vi "ObtainCmdQueue.vi"(0 "queueName":string="default", 11 "error in (no error)":errorcluster) -> (4 "cmdRef":T1, 15 "error out":errorcluster)   [LabVIEW 2017, in "vsws.lvlib"]
uses:
  vsws.lvlib
  cmdRef.ctl
  cmd.ctl
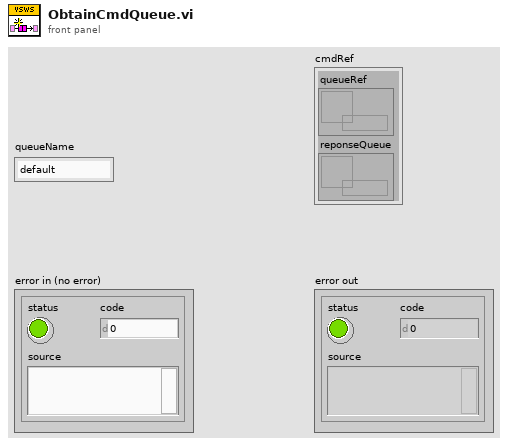
[diagram p1: front panel]
types:
  T1 = typedef "vsws.lvlib/cmdRef.ctl" = cluster{"queueRef":refnum<queue>, "reponseQueue":refnum<queue>}
  T2 = typedef "vsws.lvlib/cmd.ctl" = cluster{"postdata":string, "reponseQueue":refnum<queue>}
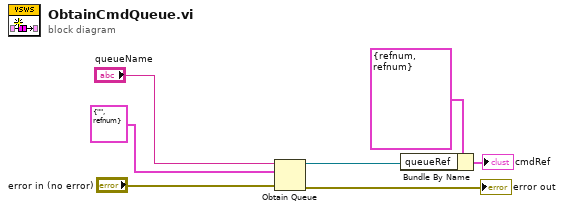
[diagram p0: block diagram]
diagram:
  n1 = Obtain Queue(name (unnamed)="queueName", element data type=T2 {"postdata"="", "reponseQueue"=refnum} ("cmd"), error in (no error)="error in (no error)") -> (queue out=w2:refnum<queue>, error out=→"error out":errorcluster)  [unwired: 2 in, 1 out]
  n2 = Bundle By Name(cluster=T1 {"queueRef"=refnum, "reponseQueue"=refnum} ("cmdRef"), "queueRef"=w2) -> (→"cmdRef":T1)
